vi "Write Timeout.vi"(8 "error in (no error)":errorcluster, 10 "Timeout":i32, 11 "Socket Communication in":refnum<class "Socket Communication.lvclass">) -> (0 "error out":errorcluster, 3 "Socket Communication out":refnum<class "Socket Communication.lvclass">)   [LabVIEW 2016, in "Socket Communication.lvclass"]
uses:
  Socket Communication.lvclass
  Socket Communication.lvclass/Socket Communication.ctl
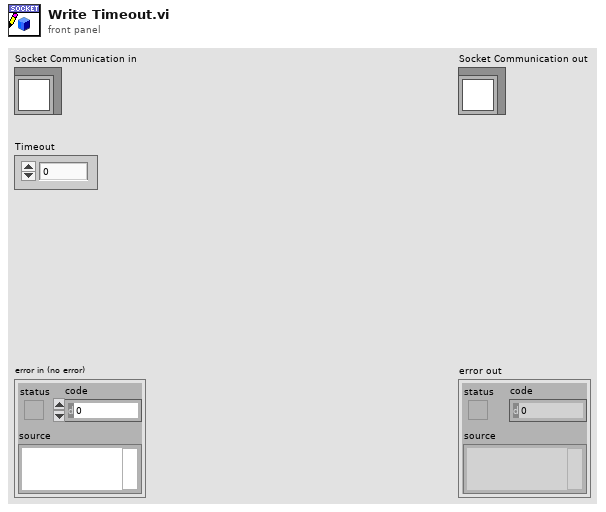
[diagram p1: front panel]
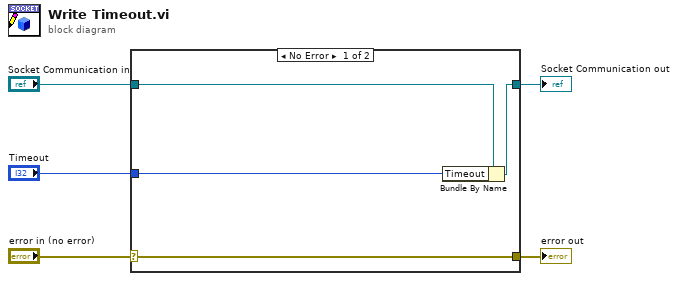
[diagram p0: block diagram]
diagram:
  n1 = case shown="No Error" "error in (no error)" {
    selector: "error in (no error)" -> [w9 w10]
    tunnel: [w9 w10] -> w4
    tunnel: [w7 w11] -> w2
    tunnel: "Socket Communication in" -> [w8 w11]
    tunnel: "Timeout" -> [w6 _]
    frame No Error {
      n2 = Bundle By Name(cluster=w8, "Timeout"=w6) -> (w7:refnum<class "Socket Communication.lvclass">)
    }
    frame Error {
    }
  }
  "error out" <- w4
  "Socket Communication out" <- w2
